vi "gyro -- launch async pll.vi"(11 "pll event pair":T1) -> (2 "reference out":refnum<vi>)   [LabVIEW 2018]
uses:
  server talkback message type.ctl
  server talkto message type.ctl
  server talk-to-back pair.ctl
panel:
  in  "set step !":dbl(slide)=7372.340425531916 min=0.0 max=16000.0 scale=0.0..16500.0 scale format="%^#6_6g"
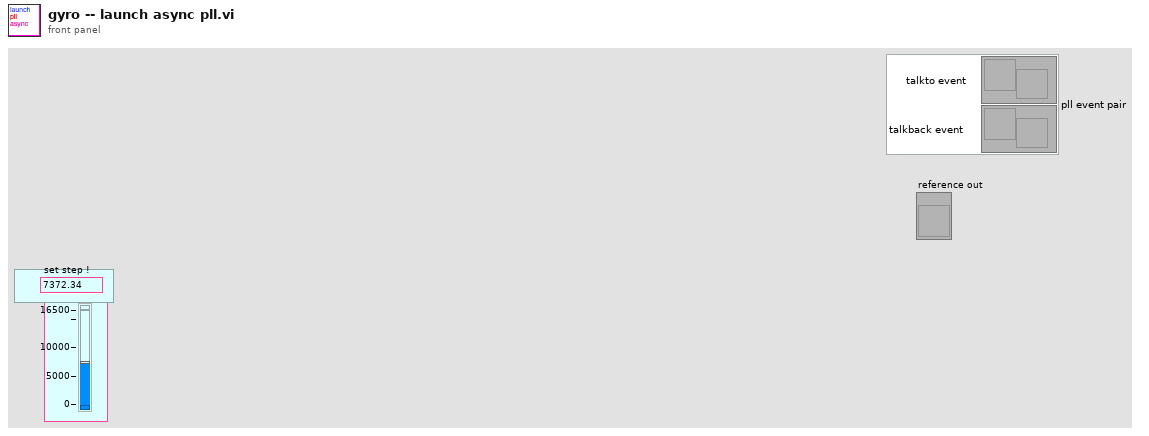
[diagram p1: front panel]
types:
  T1 = typedef "server talk-to-back pair.ctl" = cluster{"talkback event":refnum<user-event>, "talkto event":refnum<user-event>}
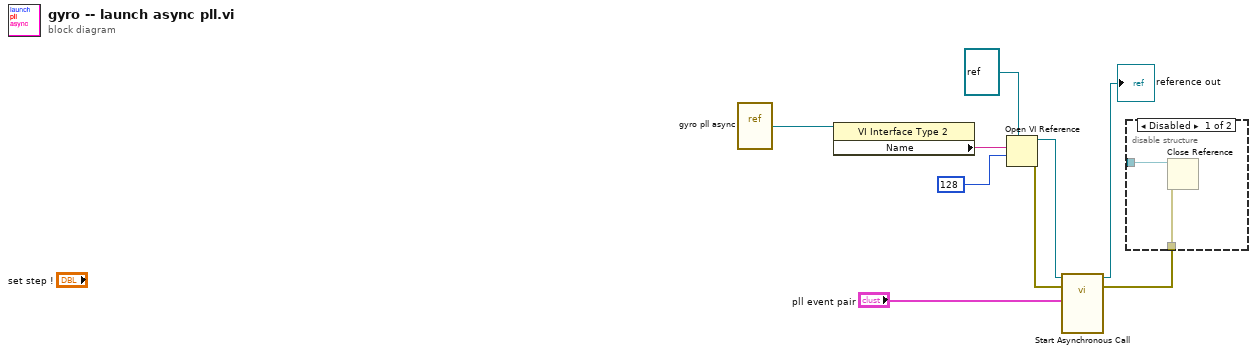
[diagram p0: block diagram]
diagram:
  n1 = vi-ref "gyro pll async.vi"() -> (w8:refnum<vi>)
  n2 = property class="VI Interface Type 2"(reference=w8) -> ("Name"=w7:string)  [unwired: 1 in, 2 out]
  n3 = Open VI Reference(type specifier VI Refnum (for type only)=refnum<vi> refnum, vi path=w7, options=128) -> (vi reference=w3:refnum<vi>, error out=w2:errorcluster)  [unwired: 3 in]
  n4 = call-by-ref "Start Asynchronous Call"(reference=w3, error in=w2, "pll event pair"="pll event pair") -> (reference out=→"reference out":refnum<vi>, error out=w5:errorcluster)  [unwired: 11 in]
  n5 = disable-structure shown="Disabled" {
    disable-tunnel: w5 -> [w11 _]
    disable-tunnel: _ -> [w10 _]
    frame Disabled {
      n6 = Close Reference(reference=w10, error in (no error)=w11) -> ()  [unwired: 1 out]
    }
    frame Enabled {
    }
  }
